vi "ReadTs530a.vi"(11 "CONFIGURATION CLUSTER":T1) -> (1 "HEATER CURRENT":dbl format="%^_2e", 2 "HEATER VOLTAGE":dbl format="%^_2e", 3 "UNMODIFIED CONFIGURATION CLUSTER":T1, 4 "HEATER POWER":dbl format="%^_2e", 5 "ANALOG SET POINT":dbl format="%_5g")   [LabVIEW 2012]
doc: "Reads the set point and heater voltage\nand current from TS-530A. Can be\nused only when AVS-47B is in remote \nmode."
panel:
  # "ReadTs530a.vi"
  # "This VI can be run only when the AVS-47B is in remote mode.  If  the bridge is in local mode,  \nall four outputs will zero. The VI does not modify the configuration cluster in any way.\n\nThis VI makes use of the fact that the A/D converter in the resistance bridge can measure the\ntemperature controller's analog set point, heater voltage and heater current. Measuring them\nis a slow process.  After the three measurements, the VI returns those three values and additionally \ncalculates the true dissipated heater power I*V. \n\nNote that the measured analog set point can deviate from its previously programmed value\nby some hundred microvolts because both the D/A converter in the TS-530A and the \nA/D converter in the AVS-47B have finite accuracy."
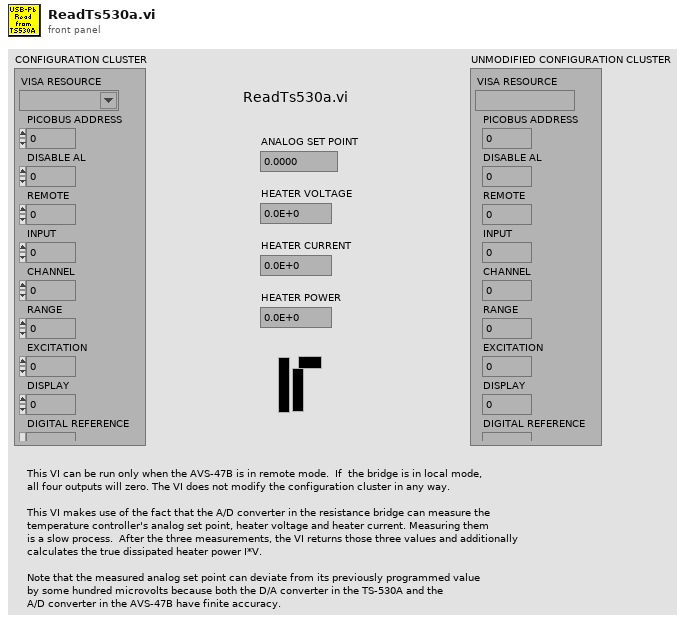
[diagram p1: front panel]
types:
  T1 = cluster{"VISA RESOURCE":refnum<visa-resource-name>, "PICOBUS ADDRESS":u8, "DISABLE AL":u8, "REMOTE":u8, "INPUT":u8, "CHANNEL":u8, "RANGE":u8, "EXCITATION":u8, "DISPLAY":u8, "DIGITAL REFERENCE":u16, "SET POINT":dbl, "PROP GAIN":u8, "INTG":u8, "DERIV":u8, "POWER BIAS":u8, "POWER RANGE":u8, "INFO STRING":string, "HEATER RESISTANCE":dbl, "INTERVAL":u8, " SENSOR dR/dT":u8}
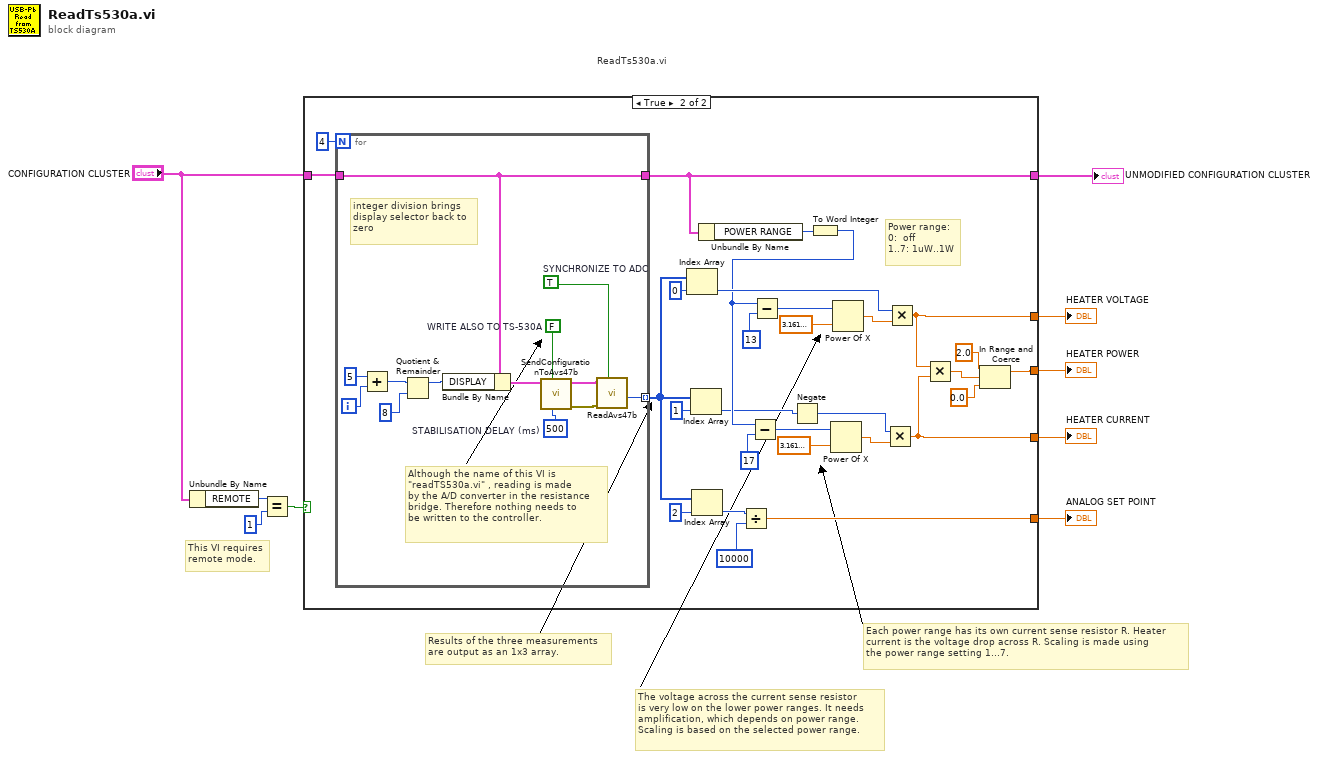
[diagram p0: block diagram]
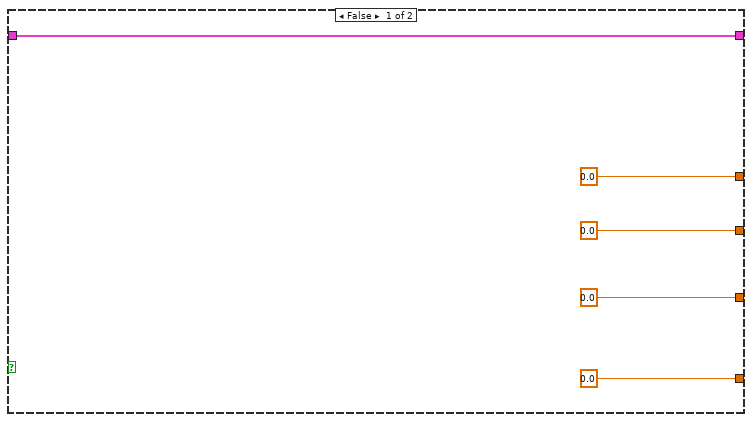
[diagram p2: hidden frame]
diagram:
  # "The voltage across the current sense resistor\nis very low on the lower power ranges. It needs\namplification, which depends on power range.\nScaling is based on the selected power range."
  # "Results of the three measurements\nare output as an 1x3 array."
  # "Each power range has its own current sense resistor R. Heater\ncurrent is the voltage drop across R. Scaling is made using\nthe power range setting 1...7."
  # "ReadTs530a.vi"
  # "This VI requires\nremote mode."
  n1 = Unbundle By Name("CONFIGURATION CLUSTER") -> ("REMOTE"=w8:u8)
  n2 = Equal?(x=w8, y=u8 1) -> (x = y?=w7:bool)
  n3 = case shown="True" w7 {
    tunnel: "CONFIGURATION CLUSTER" -> [w14 w42]
    tunnel: [w14 w15] -> w1
    tunnel: [sgl 0.0 w22] -> w3
    tunnel: [sgl 0.0 w19] -> w4
    tunnel: [sgl 0.0 w21] -> w5
    tunnel: [0.0 w20] -> w6
    frame False {
    }
    frame True {
      # "Power range:\n0:  off\n1..7: 1uW..1W"
      n4 = for {
        N: 4 -> [_]
        tunnel: w42 -> [w52]
        tunnel: [w52] -> w15
        tunnel: [w48] -> w38 mode=indexing
        i -> [w53]
        w51 = 500  # STABILISATION DELAY (ms)
        w47 = TRUE  # SYNCHRONIZE TO ADC
        w55 = FALSE  # WRITE ALSO TO TS-530A
        # "integer division brings\ndisplay selector back to\nzero"
        # "Although the name of this VI is \n\"readTS530a.vi\" , reading is made\nby the A/D converter in the resistance\nbridge. Therefore nothing needs to \nbe written to the controller."
        n5 = Add(x=5 ("y"), y=w53) -> (x+y=w46:i32)
        n6 = Quotient & Remainder(x=w46, y=8) -> (x-y*floor(x/y)=w45:i32)  [unwired: 1 out]
        n7 = Bundle By Name(cluster=w52, "DISPLAY"=w45) -> (w56:T1)
        n8 = call "SendConfigurationToAvs47b.vi"("STABILISATION DELAY (ms)"=w51, "WRITE ALSO TO TS-530A"=w55, "CONFIGURATION CLUSTER"=w56) -> ("LV ERROR OUT"=w50:errorcluster, "UNMODIFIED CONFIGURATION CLUSTER"=w49:T1)  [unwired: 5 in, 2 out]
        n9 = call "ReadAvs47b.vi"("SYNCHRONISE TO ADC"=w47, "LV ERROR IN"=w50, "CONFIGURATION CLUSTER"=w49) -> ("ADC"=w48:i32)  [unwired: 3 in, 5 out]
      }
      n10 = Index Array(array=w38, index=0) -> (element=w30:i32)
      n11 = Index Array(array=w38, index=1) -> (element=w24:i32)
      n12 = Index Array(array=w38, index=2) -> (element=w37:i32)
      n13 = Unbundle By Name(w15) -> ("POWER RANGE"=w33:u8)
      n14 = Divide(x=w37, y=10000) -> (x/y=w20:dbl)
      n15 = Negate(x=w24) -> (-x=w23:i32)
      n16 = To Word Integer(number=w33) -> (16bit integer=w25:i16)
      n17 = Subtract(x=w25, y=u8 17) -> (x-y=w28:i16)
      n18 = Subtract(x=w25, y=u8 13) -> (x-y=w34:i16)
      n19 = Power Of X(1:sgl 3.162 ("x"), 2:w28) -> (0:w26:sgl)
      n20 = Power Of X(1:sgl 3.162 ("x"), 2:w34) -> (0:w31:sgl)
      n21 = Multiply(x=w23, y=w26) -> (x*y=w21:sgl)
      n22 = Multiply(x=w30, y=w31) -> (x*y=w22:sgl)
      n23 = Multiply(x=w22, y=w21) -> (x*y=w17:sgl)
      n24 = In Range and Coerce(upper limit=sgl 2.0 ("lower limit"), x=w17, lower limit=sgl 0.0) -> (coerced(x)=w19:sgl)  [unwired: 1 out]
    }
  }
  "HEATER VOLTAGE" <- w3
  "HEATER POWER" <- w4
  "HEATER CURRENT" <- w5
  "ANALOG SET POINT" <- w6
  "UNMODIFIED CONFIGURATION CLUSTER" <- w1
